vi "TakeSampleCalibrationImages.vi"(6 "ExposureTime_us":u32, 7 "TLCamera reference in":refnum<k24>, 8 "Error In":errorcluster, 9 "Img2 in":T1, 10 "Img1 in":T1, 11 "MotorController in":refnum<class "MotorController.lvclass">) -> (0 "Error Out":errorcluster, 1 "Img2 out":T1, 2 "Img1 out":T1, 3 "MotorController out":refnum<class "MotorController.lvclass">, 5 "TLCamera reference out":refnum<k24>)   [LabVIEW 2019]
uses:
  MotorController.lvclass
  <vilib>/vision/Image Controls.llb/IMAQ Image.ctl
  C:/Users/jleeman/git_repos/CAxis_Machine/C-Axis LabView Controller/Library_X64/Thorlabs.TSI.TLCameraInterfaces.dll
  Library_X64/Thorlabs.TSI.TLCameraInterfaces.dll
  Axes_enum_typedef.ctl
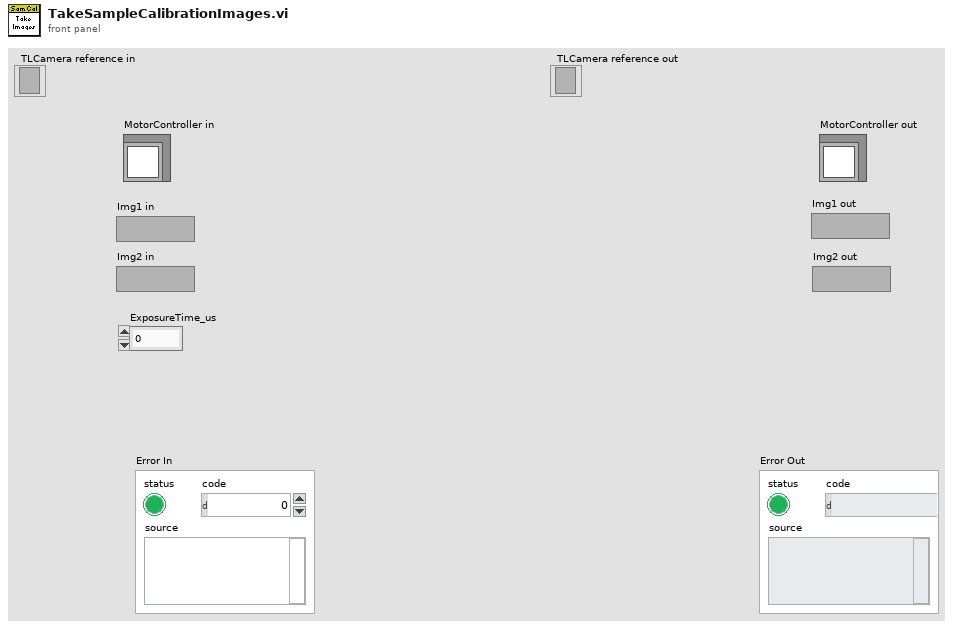
[diagram p1: front panel]
types:
  T1 = typedef "IMAQ Image.ctl" = refnum<image>
  T2 = typedef "Axes_enum_typedef.ctl" = enum16{"Polarizer 1", "Polarizer 2", "Sample", "Stage"}
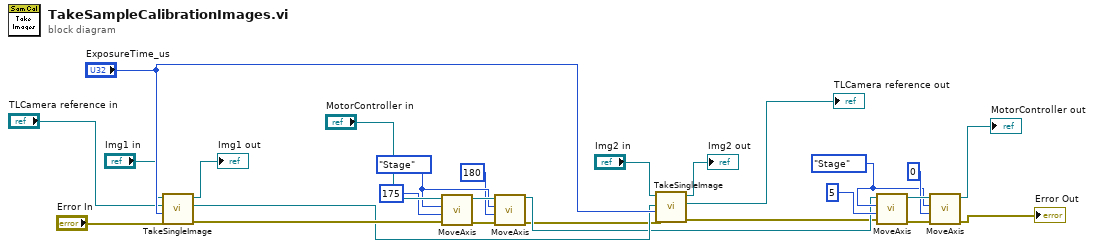
[diagram p0: block diagram]
diagram:
  w6 = Axes_enum_typedef."Stage" ("Axis")
  w13 = Axes_enum_typedef."Stage" ("Axis")
  n1 = call "TakeSingleImage.vi"("Image"="Img1 in", "TLCamera reference in"="TLCamera reference in", "ExposureTime_us"="ExposureTime_us", "Error In"="Error In") -> ("Image Out"=→"Img1 out":T1, "TLCamera reference out"=w18:refnum<k24>, "Error Out"=w23:errorcluster)  [unwired: 4 in]
  n2 = call "MoveAxis.vi"("error in (no error)"=w23, "Position"=u16 175, "Axis"=w13, "MotorController in"="MotorController in") -> ("error out"=w15:errorcluster, "MotorController out"=w14:refnum<class "MotorController.lvclass">)  [unwired: 6 in]
  n3 = call "MoveAxis.vi"("error in (no error)"=w15, "Position"=u16 180, "Axis"=w13, "MotorController in"=w14) -> ("error out"=w4:errorcluster, "MotorController out"=w5:refnum<class "MotorController.lvclass">)  [unwired: 6 in]
  n4 = call "TakeSingleImage.vi"("Image"="Img2 in", "TLCamera reference in"=w18, "ExposureTime_us"="ExposureTime_us", "Error In"=w4) -> ("Image Out"=→"Img2 out":T1, "TLCamera reference out"=→"TLCamera reference out":refnum<k24>, "Error Out"=w3:errorcluster)  [unwired: 4 in]
  n5 = call "MoveAxis.vi"("error in (no error)"=w3, "Position"=u16 5, "Axis"=w6, "MotorController in"=w5) -> ("error out"=w10:errorcluster, "MotorController out"=w9:refnum<class "MotorController.lvclass">)  [unwired: 6 in]
  n6 = call "MoveAxis.vi"("error in (no error)"=w10, "Position"=u16 0, "Axis"=w6, "MotorController in"=w9) -> ("error out"=→"Error Out":errorcluster, "MotorController out"=→"MotorController out":refnum<class "MotorController.lvclass">)  [unwired: 6 in]
